vi "Defer Panel Updates.vi"(8 "error in":errorcluster, 10 "Defer Panel Updates":bool=TRUE, 11 "VI in":refnum<vi>) -> (0 "error out":errorcluster)   [LabVIEW 2020, in "Panther Dashboard.lvlib"]
uses:
  Panther Dashboard.lvlib
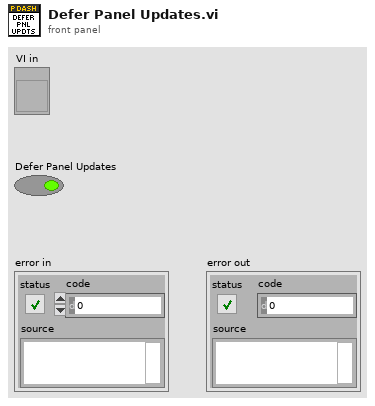
[diagram p1: front panel]
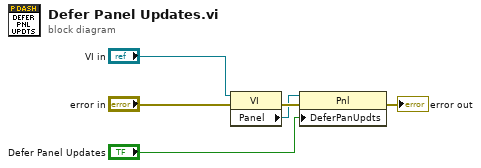
[diagram p0: block diagram]
diagram:
  n1 = property class="VI"(reference="VI in", error in="error in") -> (error out=w4:errorcluster, "Panel"=w3:refnum<vi>)  [unwired: 1 out]
  n2 = property class="Pnl"(reference=w3, error in=w4, "DeferPanUpdts"="Defer Panel Updates") -> (error out=→"error out":errorcluster)  [unwired: 1 out]
